vi "fpga_I32xU32 Multiplier (MSBs).vi"(1 "y[U32]":u32, 2 "x[I32]":i32) -> (0 "x*y[I32 MSB]":i32)   [LabVIEW 2011, in "NI_EP_Resample_FPGA.lvlib"]
uses:
  <vilib>/rvi/Arithmetic/AddSubMult/XNode/nirviSatArithmetic.xnode
  <vilib>/addons/Electrical Power/PQ/Resampling/NI_EP_Resample_FPGA.lvlib
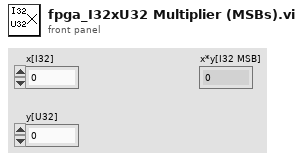
[diagram p1: front panel]
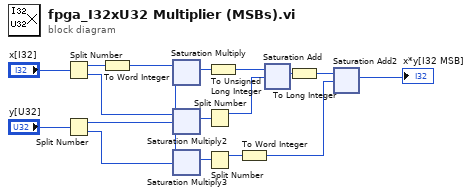
[diagram p0: block diagram]
diagram:
  n1 = Split Number(x="x[I32]") -> (hi(x)=w9:u16, lo(x)=w14:u16)
  n2 = Split Number(x="y[U32]") -> (hi(x)=w12:u16, lo(x)=w11:u16)
  n3 = To Word Integer(number=w9) -> (16bit integer=w6:i16)
  n4 = xnode ("Saturation Multiply")("x"=w6, "y"=w12) -> ("x*y"=w4:i32)
  n5 = xnode ("Saturation Multiply2")("x"=w14, "y"=w12) -> ("x*y"=w15:u32)
  n6 = xnode ("Saturation Multiply3")("x"=w6, "y"=w11) -> ("x*y"=w10:i32)
  n7 = Split Number(x=w15) -> (hi(x)=w16:u16)  [unwired: 1 out]
  n8 = Split Number(x=w10) -> (hi(x)=w7:u16)  [unwired: 1 out]
  n9 = To Unsigned Long Integer(number=w4) -> (unsigned 32bit integer=w3:u32)
  n10 = To Word Integer(number=w7) -> (16bit integer=w5:i16)
  n11 = xnode ("Saturation Add")("x"=w3, "y"=w16) -> ("x+y"=w8:u32)
  n12 = To Long Integer(number=w8) -> (32bit integer=w2:i32)
  n13 = xnode ("Saturation Add2")("x"=w2, "y"=w5) -> ("x+y"=→"x*y[I32 MSB]":i32)
